vi "Tektronix TDS 200 1000 2000 Series Edge Triggered Acquisition.vi"() -> ()   [LabVIEW 2012]
doc: "This example shows how to configure the oscilloscope to perform an edge-triggered waveform acquisition."
uses:
  <instrlib>/Tektronix TDS 200 1000 2000 Series/Public/Configure/Configure Trigger (Edge).vi
  <instrlib>/Tektronix TDS 200 1000 2000 Series/Public/Data/Read (Single Waveform).vi
  <instrlib>/Tektronix TDS 200 1000 2000 Series/Tektronix TDS 200 1000 2000 Series.lvlib
panel:
  in  "Channel (0: Channel 1)":u16(ring) items=["Channel 1", "Channel 2", "Channel 3", "Channel 4", "Math", "Reference A", "Reference B", "Reference C", "Reference D"]
  in  "Serial Configuration":T1={"Baud Rate"=9600, "Parity"=0, "Stop Bits"=10, "Flow Control"=0} {"Flow Control" items=["None", "XON/XOFF", "RTS/CTS", "XON/XOFF & RTS/CTS", "DTR/DSR", "XON/XOFF & DTR/DSR"]; "Stop Bits" items=["1.0"=10, "1.5"=15, "2.0"=20]; "Parity" items=["None", "Odd", "Even", "Mark", "Space"]; "Baud Rate" items=["300"=300, "600"=600, "1200"=1200, "2400"=2400, "4800"=4800, "9600"=9600, "19200"=19200]}
  in  "Vertical Coupling (1: DC)":u16(ring)=1 items=["AC", "DC", "Ground"]
  in  "Probe Attenuation (1.0)":dbl=1.0
  in  "Trigger Level (0.0 V)":dbl
  out "Waveform Data":waveform(dbl)(graph)
  in  "VISA resource name":refnum<visa-resource-name>
  # "(C) 2009-2014 National Instruments.  ALL RIGHTS RESERVED."
  # "To change Vertical Range and Timebase settings, \nplease modify constants on the Block Diagram"
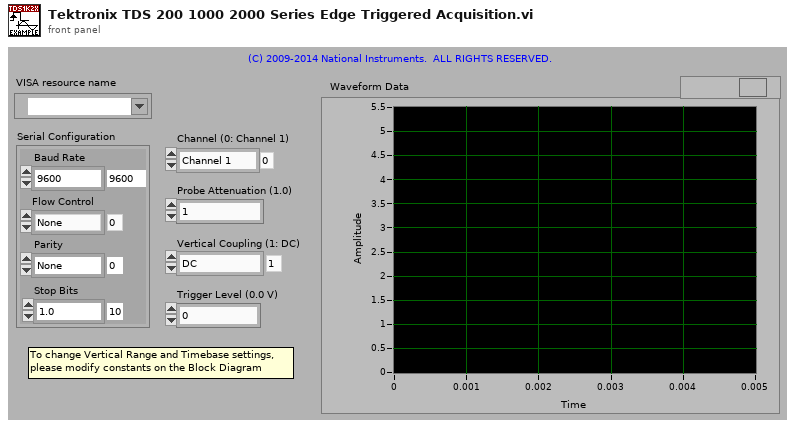
[diagram p1: front panel]
types:
  T1 = cluster{"Baud Rate":u32, "Parity":u16, "Stop Bits":u16, "Flow Control":u16}
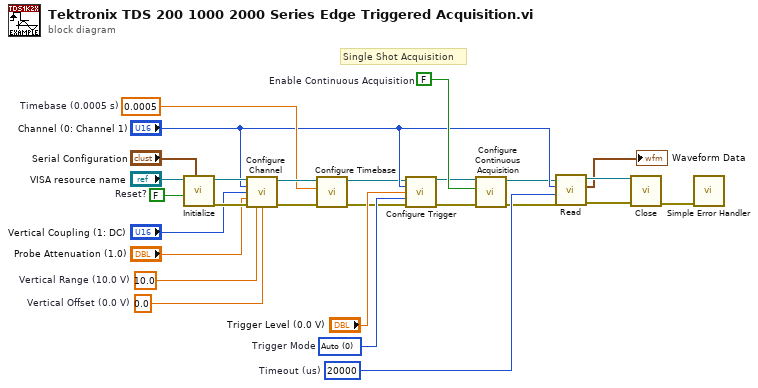
[diagram p0: block diagram]
diagram:
  w8 = u16 0 items=["Auto", "Normal"]  # Trigger Mode
  w9 = FALSE  # Reset?
  w12 = 0.0  # Vertical Offset (0.0 V)
  w24 = 0.0005  # Timebase (0.0005 s)
  w17 = 10.0  # Vertical Range (10.0 V)
  w3 = u32 20000  # Timeout (us)
  w16 = FALSE  # Enable Continuous Acquisition
  # "Single Shot Acquisition"
  n1 = call <instrlib>:"Initialize.vi"("Serial Configuration"="Serial Configuration", "Reset? (T: Yes)"=w9, "VISA resource name"="VISA resource name") -> ("error out"=w21:errorcluster, "VISA resource name out"=w22:refnum<visa-resource-name>)  [unwired: 2 in, 5 out]
  n2 = call <instrlib>:"Configure Channel.vi"("VISA resource name"=w22, "Channel (0: Channel 1)"="Channel (0: Channel 1)", "Vertical Coupling (1: DC)"="Vertical Coupling (1: DC)", "Probe Attenuation (10: 10X)"="Probe Attenuation (1.0)", "error in (no error)"=w21, "Vertical Range (10.0 V/div)"=w17, "Vertical Offset (0.0 divs)"=w12) -> ("VISA resource name out"=w25:refnum<visa-resource-name>, "error out"=w26:errorcluster)  [unwired: 2 in, 5 out]
  n3 = call <instrlib>:"Configure Timebase.vi"("error in (no error)"=w26, "Timebase (0.0005 s)"=w24, "VISA resource name"=w25) -> ("error out"=w6:errorcluster, "VISA resource name out"=w7:refnum<visa-resource-name>)  [unwired: 1 in, 6 out]
  n4 = call-poly <instrlib>:"Configure Trigger.vi"("VISA resource name"=w7, "Trigger Source (0: Channel 1)"="Channel (0: Channel 1)", "Trigger Level (0.0 V)"="Trigger Level (0.0 V)", "Trigger Mode (0: Auto)"=w8, "error in (no error)"=w6) -> ("VISA resource name out"=w5:refnum<visa-resource-name>, "error out"=w4:errorcluster)  [unwired: 2 in, 7 out]
  n5 = call <instrlib>:"Configure Continuous Acquisition.vi"("error in (no error)"=w4, "Enable Continuous Acquisition Mode (True)"=w16, "VISA resource name"=w5) -> ("error out"=w1:errorcluster, "VISA resource name out"=w2:refnum<visa-resource-name>)  [unwired: 7 out]
  n6 = call-poly <instrlib>:"Read.vi"("error in (no error)"=w1, "Timeout (10000 ms)"=w3, "Source (0: Channel 1)"="Channel (0: Channel 1)", "VISA resource name"=w2) -> ("error out"=w19:errorcluster, "Waveform Data"=→"Waveform Data":waveform(dbl), "VISA resource name out"=w20:refnum<visa-resource-name>)  [unwired: 5 out]
  n7 = call <instrlib>:"Close.vi"("error in (no error)"=w19, "VISA resource name"=w20) -> ("error out"=w27:errorcluster)  [unwired: 9 out]
  n8 = call <vilib>:"Simple Error Handler.vi"("error in (no error)"=w27) -> ()  [unwired: 1 in, 8 out]
